vi "Update Selected Script.vi"(8 "error in":errorcluster, 10 "Script UI Ctrl Ref":T2, 11 "Script Meas Config Ctrl Ref":T1) -> (0 "error out":errorcluster)   [LabVIEW 2025, in "Fgen Script Mode UI.lvlib"]
uses:
  Fgen Script Mode UI.lvlib
  Typedef/Script UI Ctrl Ref.ctl
  Typedef/Script Meas Config Ctrl Ref.ctl
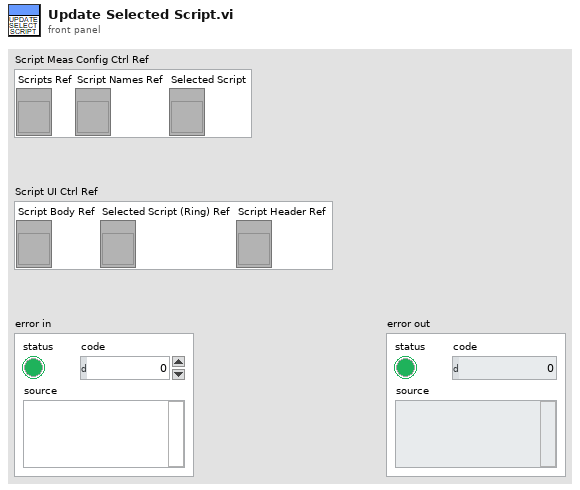
[diagram p1: front panel]
types:
  T1 = typedef "Fgen Script Mode UI.lvlib/Script Meas Config Ctrl Ref.ctl" = cluster{"Scripts Ref":refnum<vi>, "Script Names Ref":refnum<vi>, "Selected Script":refnum<vi>}
  T2 = typedef "Fgen Script Mode UI.lvlib/Script UI Ctrl Ref.ctl" = cluster{"Script Body Ref":refnum<vi>, "Selected Script (Ring) Ref":refnum<vi>, "Script Header Ref":refnum<vi>}
  T3 = enum8{"Enabled", "Disabled", "Disabled and Grayed Out"}
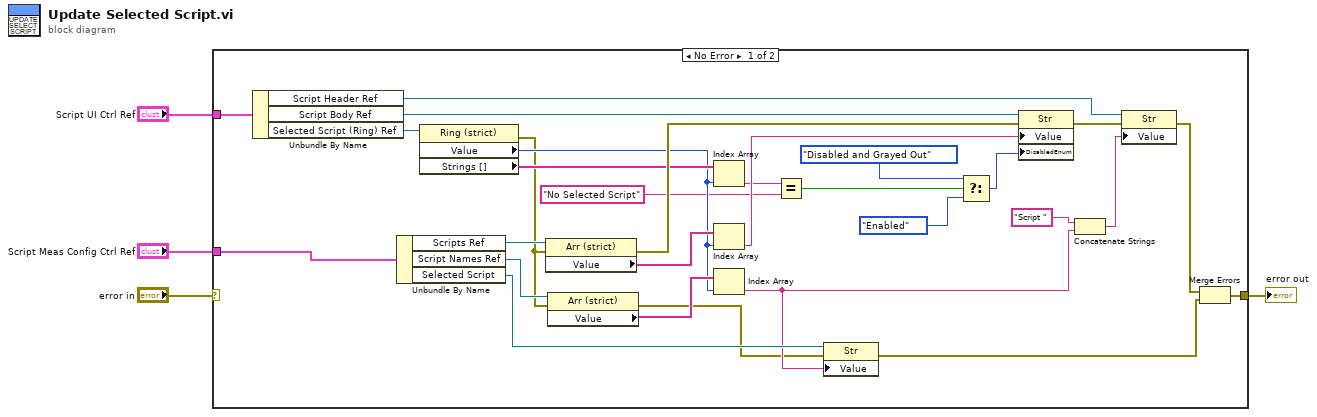
[diagram p0: block diagram]
diagram:
  n1 = case shown="No Error" "error in" {
    selector: "error in" -> [_ w34]
    tunnel: [w7 w34] -> w3
    tunnel: "Script Meas Config Ctrl Ref" -> [w31 _]
    tunnel: "Script UI Ctrl Ref" -> [w33 _]
    frame No Error {
      n2 = Unbundle By Name(w33) -> ("Script Header Ref"=w22:refnum<vi>, "Script Body Ref"=w29:refnum<vi>, "Selected Script (Ring) Ref"=w32:refnum<vi>)
      n3 = Unbundle By Name(w31) -> ("Scripts Ref"=w30:refnum<vi>, "Script Names Ref"=w25:refnum<vi>, "Selected Script"=w10:refnum<vi>)
      n4 = property class="Ring (strict)"(reference=w32) -> (error out=w8:errorcluster, "Value"=w17:u16, "Strings []"=w18:string[])  [unwired: 1 in, 1 out]
      n5 = property class="Arr (strict)"(reference=w30, error in=w8) -> (error out=w27:errorcluster, "Value"=w19:string[])  [unwired: 1 out]
      n6 = property class="Arr (strict)"(reference=w25, error in=w8) -> (error out=w5:errorcluster, "Value"=w24:string[])  [unwired: 1 out]
      n7 = Index Array(array=w18, index=w17) -> (element=w16:string)
      n8 = Index Array(array=w19, index=w17) -> (element=w28:string)
      n9 = Index Array(array=w24, index=w17) -> (element=w9:string)
      n10 = Equal?(x=w16, y="No Selected Script" ("Scripts Array")) -> (x = y?=w14:bool)
      n11 = property class="Str"(reference=w10, error in=w5, "Value"=w9) -> (error out=w6:errorcluster)  [unwired: 1 out]
      n12 = Select(t=T3."Disabled and Grayed Out" ("Disabled"), s=w14, f=T3."Enabled" ("Disabled")) -> (s? t:f=w11:T3)
      n13 = property class="Str"(reference=w29, error in=w27, "Value"=w28, "DisabledEnum"=w11) -> (error out=w26:errorcluster)  [unwired: 1 out]
      n14 = Concatenate Strings("Script " ("string"), w9) -> (w20:string)
      n15 = property class="Str"(reference=w22, error in=w26, "Value"=w20) -> (error out=w23:errorcluster)  [unwired: 1 out]
      n16 = Merge Errors(w23, w6) -> (w7:errorcluster)
    }
    frame Error {
    }
  }
  "error out" <- w3
